vi "GetText.vi"(8 "error in":errorcluster, 11 "Switch Insrument in":refnum<class "Switch Instrument.lvclass">) -> (0 "error out":errorcluster, 1 "additional text":string, 2 "text":string, 3 "Switch Instrument out":refnum<class "Switch Instrument.lvclass">, 4 "glyph":string)   [LabVIEW 2025, in "Switch.lvlib" / "Switch Instrument.lvclass"]
doc: "Copyright 2017 National Instruments Corporation\n\nLicensed under the Apache License, Version 2.0 (the \"License\"); you may not use this file except in compliance with the License. You may obtain a copy of the License at http://www.apache.org/licenses/LICENSE-2.0\nUnless required by applicable law or agreed to in writing, software distributed under the License is distributed on an \"AS IS\" BASIS, WITHOUT WARRANTIES OR CONDITIONS OF ANY KIND, either express or implied. See the License for the specific language governing permissions and limitations under the License."
uses:
  Switch Instrument.lvclass
  Switch Instrument.lvclass/Switch Instrument.ctl
  Switch configuration/Switch configuration.lvclass
  C:/Users/Public/Documents/Sandia National Labs/TSS Plugin/Abstract Engine.lvlibp/Instrument configuration/Instrument configuration.lvclass
  Users/Public/Documents/Sandia National Labs/TSS Plugin/Abstract Engine.lvlibp/Instrument configuration/Read Instrument Setting.vi
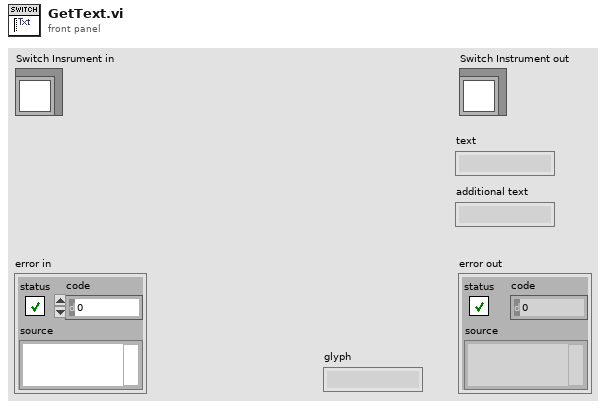
[diagram p1: front panel]
types:
  T1 = typedef "Abstract Engine.lvlibp/Instrument configuration.lvclass/Default Instrument.ctl" = cluster{"Type":string, "Address":string, "SW Alias":string, "Description":string, "Enabled":bool}
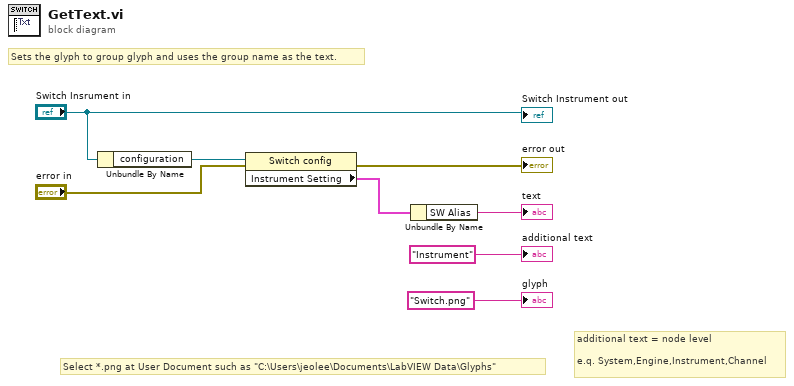
[diagram p0: block diagram]
diagram:
  # "Select *.png at User Document such as \"C:\\Users\\jeolee\\Documents\\LabVIEW Data\\Glyphs\""
  # "additional text = node level\n\ne.q. System,Engine,Instrument,Channel"
  # "Sets the glyph to group glyph and uses the group name as the text."
  n1 = Unbundle By Name("Switch Insrument in") -> ("configuration"=w2:refnum<class "Switch configuration.lvclass">)
  n2 = property class="Switch config"(reference=w2, error in="error in") -> (error out=→"error out":errorcluster, "Instrument Setting"=w1:T1)  [unwired: 1 out]
  n3 = Unbundle By Name(w1) -> ("SW Alias"=→"text":string)
  "Switch Instrument out" <- "Switch Insrument in"
  "additional text" <- "Instrument" ("additional text")
  "glyph" <- "Switch.png" ("glyph")
